vi "Copy Help.vi"(8 "Error In":errorcluster, 11 "Target Project Root In":path) -> (0 "Error Out":errorcluster, 3 "Target Project Root Out":path)   [LabVIEW 2017, in "Scripts.lvlib"]
doc: "Copies the `src\\Help` folder to the target destination. This is necessary because the Save for Previous operation does not automatically copy the `Help` folder and its contents to the target destination. The Help source is NOT included in the project file because it would be a hassle to include all of the files using virtual folders."
uses:
  Scripts.lvlib
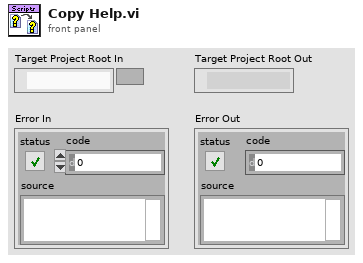
[diagram p1: front panel]
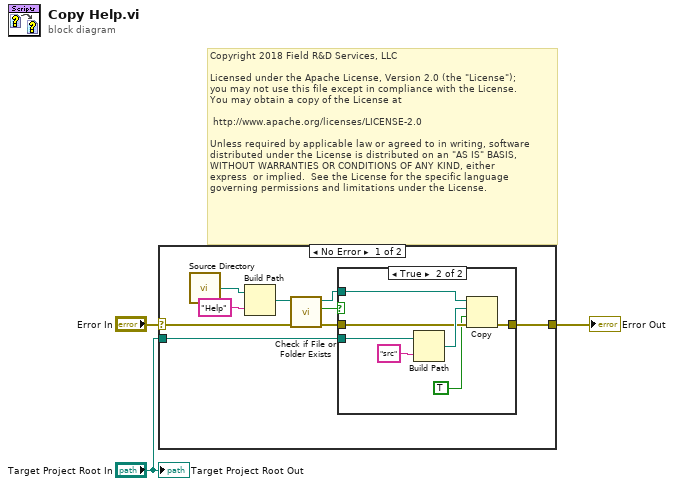
[diagram p0: block diagram]
diagram:
  # "Copyright 2018 Field R&D Services, LLC\n\nLicensed under the Apache License, Version 2.0 (the \"License\");\nyou may not use this file except in compliance with the License.\nYou may obtain a copy of the License at\n\n\thttp://www.apache.org/licenses/LICENSE-2.0\n\nUnless required by applicable law or agreed to in writing, software\ndistributed under the License is distributed on an \"AS IS\" BASIS,\nWITHOUT WARRANTIES OR CONDITIONS OF ANY KIND, either \nexpress  or implied.  See the License for the specific language \ngoverning permissions and limitations under the License."
  n1 = case shown="No Error" "Error In" {
    selector: "Error In" -> [w11 w21]
    tunnel: "Target Project Root In" -> [w4 _]
    tunnel: [w12 w21] -> w2
    frame No Error {
      n2 = call "Source Directory.vi"() -> ("Source Directory"=w8:path)
      n3 = Build Path(base path=w8, name or relative path="Help") -> (appended path=w6:path)
      n4 = call <vilib>:"Check if File or Folder Exists.vi"("error in (no error)"=w11, "path"=w6) -> ("error out"=w10:errorcluster, "file or folder exists?"=w9:bool, "dup path"=w5:path)  [unwired: 7 in]
      n5 = case shown="True" w9 {
        tunnel: w4 -> [_ w20]
        tunnel: [w13 w19] -> w12
        tunnel: w10 -> [w13 w16]
        tunnel: w5 -> [_ w14]
        frame False {
        }
        frame True {
          n6 = Build Path(base path=w20, name or relative path="src") -> (appended path=w18:path)
          n7 = Copy(8:w16, 9:TRUE ("overwrite (F)"), 10:w18, 11:w14) -> (0:w19:errorcluster)  [unwired: 1 in, 2 out]
        }
      }
    }
    frame Error {
    }
  }
  "Error Out" <- w2
  "Target Project Root Out" <- "Target Project Root In"
